vi "Plot Data.vi"(0 "Data Array":dbl[][](array[numeric]), 11 "Seconds":dbl[](array[numeric])) -> (4 "Number of Plots":i32=1, 6 "XY Plot - 1 Trace":cluster{"Seconds":dbl[], "Data Array":dbl[]}[](graph), 8 "XY Plot - 2 Traces":cluster{"Seconds":dbl[], "Data Array":dbl[]}[](graph), 10 "XY Plot - 3 Traces":cluster{"Seconds":dbl[], "Data Array":dbl[]}[](graph), 13 "XY Plot - 6 Traces":cluster{"Seconds":dbl[], "Data Array":dbl[]}[](graph), 14 "XY Plot - 5 Traces":cluster{"Seconds":dbl[], "Data Array":dbl[]}[](graph), 15 "XY Plot - 4 Traces":cluster{"Seconds":dbl[], "Data Array":dbl[]}[](graph))   [LabVIEW 2017]
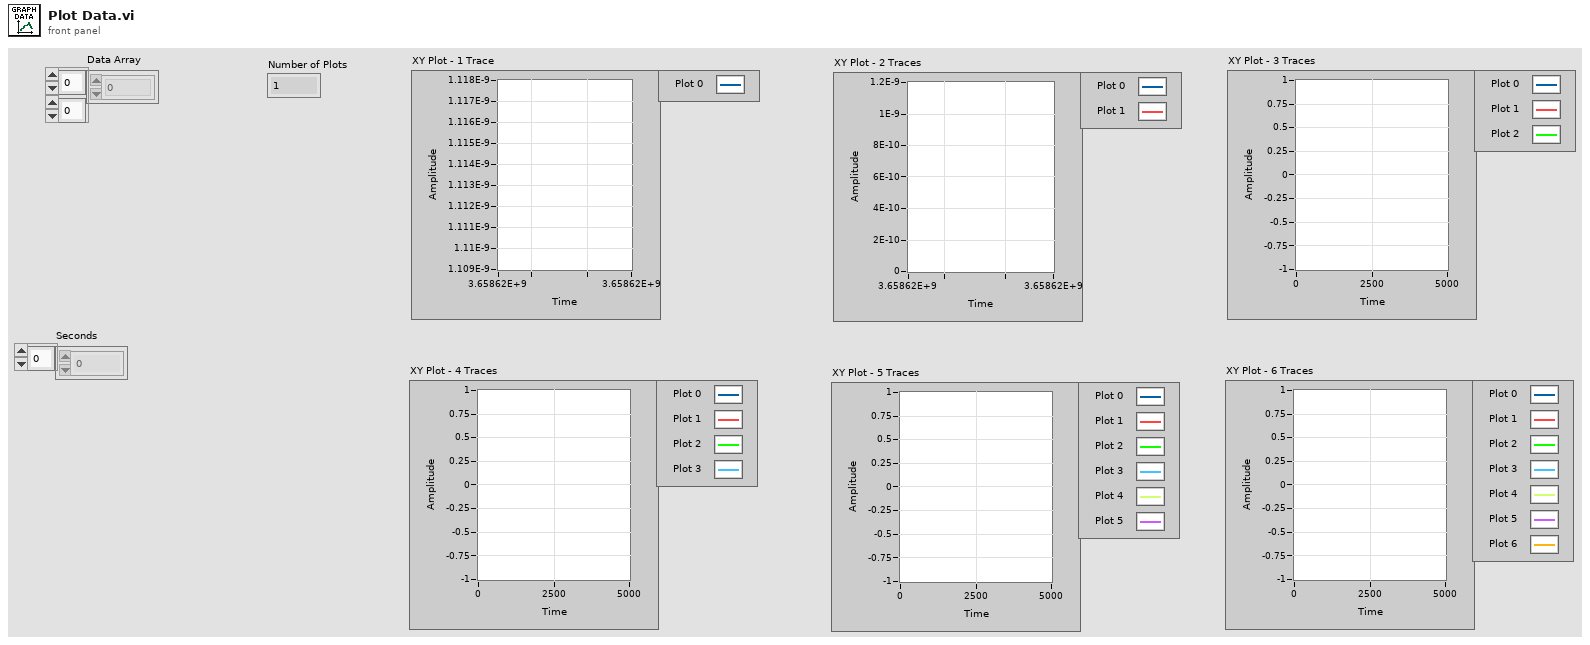
[diagram p1: front panel]
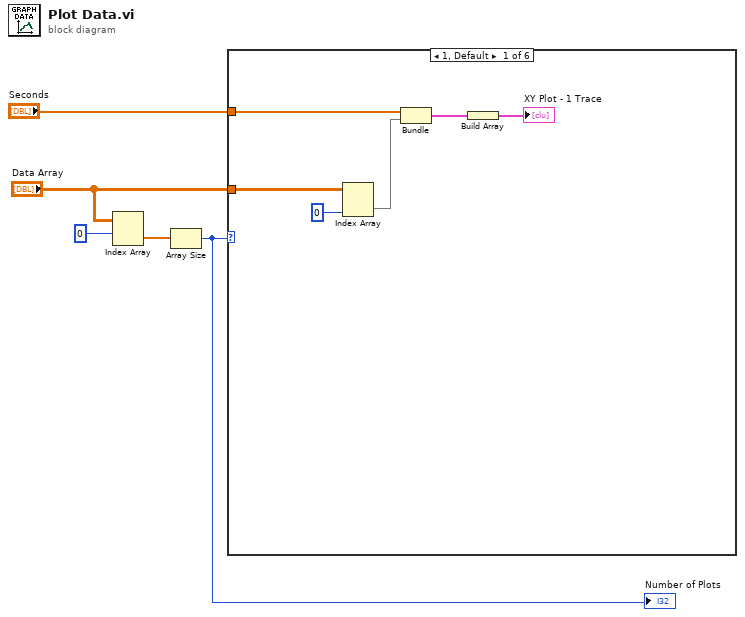
[diagram p0: block diagram]
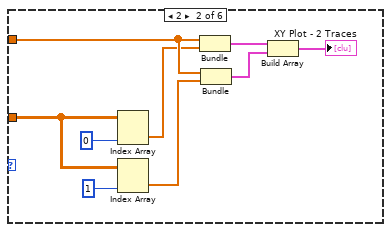
[diagram p2: hidden frame]
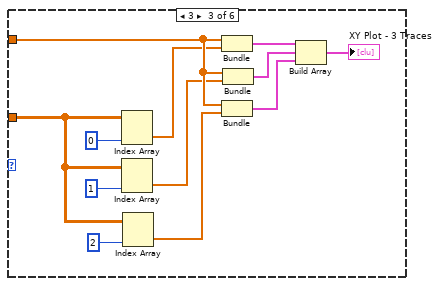
[diagram p3: hidden frame]
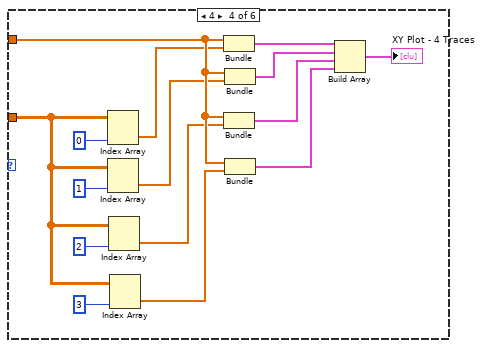
[diagram p4: hidden frame]
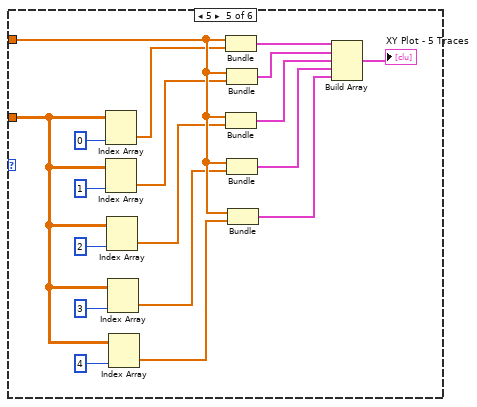
[diagram p5: hidden frame]
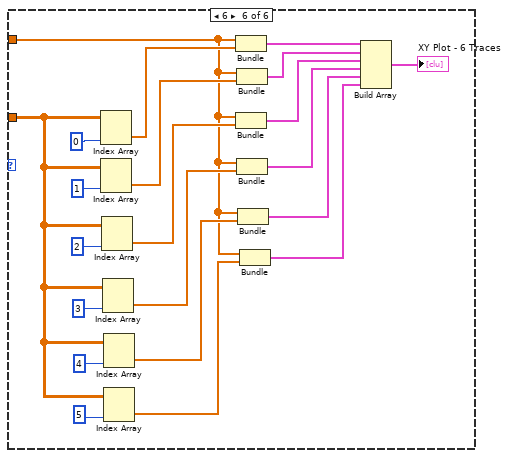
[diagram p6: hidden frame]
diagram:
  n1 = Index Array(array="Data Array", index (row)=0) -> (element=w4:dbl[])  [unwired: 1 in]
  n2 = Array Size(array=w4) -> (size(s)=w2:i32)
  "Number of Plots" <- w2
  n3 = case shown="1, Default" w2 {
    tunnel: "Seconds" -> [w11 w20 w32 w47 w65 w66]
    tunnel: "Data Array" -> [w10 w17 w25 w36 w51 w70]
    frame 1, Default {
      n4 = Index Array(array=w10, index (col)=0 ("index")) -> (element=w8:dbl[])  [unwired: 1 in]
      n5 = Bundle("Seconds"=w11, "Data Array"=w8) -> (w7:cluster{"Seconds":dbl[], "Data Array":dbl[]})  [unwired: 1 in]
      n6 = Build Array(w7) -> (→"XY Plot - 1 Trace":cluster{"Seconds":dbl[], "Data Array":dbl[]}[])
    }
    frame 2 {
      n7 = Index Array(array=w17, index (col)=0 ("index")) -> (element=w18:dbl[])  [unwired: 1 in]
      n8 = Index Array(array=w17, index (col)=1) -> (element=w15:dbl[])  [unwired: 1 in]
      n9 = Bundle("Seconds"=w20, "Data Array"=w18) -> (w14:cluster{"Seconds":dbl[], "Data Array":dbl[]})  [unwired: 1 in]
      n10 = Bundle("Seconds"=w20, "Data Array"=w15) -> (w13:cluster{"Seconds":dbl[], "Data Array":dbl[]})  [unwired: 1 in]
      n11 = Build Array(w14, w13) -> (→"XY Plot - 2 Traces":cluster{"Seconds":dbl[], "Data Array":dbl[]}[])
    }
    frame 3 {
      n12 = Index Array(array=w25, index (col)=0 ("index")) -> (element=w30:dbl[])  [unwired: 1 in]
      n13 = Index Array(array=w25, index (col)=1) -> (element=w28:dbl[])  [unwired: 1 in]
      n14 = Index Array(array=w25, index (col)=2) -> (element=w23:dbl[])  [unwired: 1 in]
      n15 = Bundle("Seconds"=w32, "Data Array"=w30) -> (w27:cluster{"Seconds":dbl[], "Data Array":dbl[]})  [unwired: 1 in]
      n16 = Bundle("Seconds"=w32, "Data Array"=w23) -> (w22:cluster{"Seconds":dbl[], "Data Array":dbl[]})  [unwired: 1 in]
      n17 = Bundle("Seconds"=w32, "Data Array"=w28) -> (w26:cluster{"Seconds":dbl[], "Data Array":dbl[]})  [unwired: 1 in]
      n18 = Build Array(w27, w26, w22) -> (→"XY Plot - 3 Traces":cluster{"Seconds":dbl[], "Data Array":dbl[]}[])
    }
    frame 4 {
      n19 = Index Array(array=w36, index (col)=0 ("index")) -> (element=w45:dbl[])  [unwired: 1 in]
      n20 = Index Array(array=w36, index (col)=1) -> (element=w43:dbl[])  [unwired: 1 in]
      n21 = Index Array(array=w36, index (col)=2) -> (element=w39:dbl[])  [unwired: 1 in]
      n22 = Index Array(array=w36, index (col)=3) -> (element=w35:dbl[])  [unwired: 1 in]
      n23 = Bundle("Seconds"=w47, "Data Array"=w45) -> (w42:cluster{"Seconds":dbl[], "Data Array":dbl[]})  [unwired: 1 in]
      n24 = Bundle("Seconds"=w47, "Data Array"=w39) -> (w38:cluster{"Seconds":dbl[], "Data Array":dbl[]})  [unwired: 1 in]
      n25 = Bundle("Seconds"=w47, "Data Array"=w43) -> (w41:cluster{"Seconds":dbl[], "Data Array":dbl[]})  [unwired: 1 in]
      n26 = Bundle("Seconds"=w47, "Data Array"=w35) -> (w34:cluster{"Seconds":dbl[], "Data Array":dbl[]})  [unwired: 1 in]
      n27 = Build Array(w42, w41, w38, w34) -> (→"XY Plot - 4 Traces":cluster{"Seconds":dbl[], "Data Array":dbl[]}[])
    }
    frame 5 {
      n28 = Index Array(array=w51, index (col)=0 ("index")) -> (element=w63:dbl[])  [unwired: 1 in]
      n29 = Index Array(array=w51, index (col)=1) -> (element=w61:dbl[])  [unwired: 1 in]
      n30 = Index Array(array=w51, index (col)=2) -> (element=w57:dbl[])  [unwired: 1 in]
      n31 = Index Array(array=w51, index (col)=3) -> (element=w54:dbl[])  [unwired: 1 in]
      n32 = Index Array(array=w51, index (col)=4) -> (element=w50:dbl[])  [unwired: 1 in]
      n33 = Bundle("Seconds"=w65, "Data Array"=w63) -> (w60:cluster{"Seconds":dbl[], "Data Array":dbl[]})  [unwired: 1 in]
      n34 = Bundle("Seconds"=w65, "Data Array"=w57) -> (w56:cluster{"Seconds":dbl[], "Data Array":dbl[]})  [unwired: 1 in]
      n35 = Bundle("Seconds"=w65, "Data Array"=w61) -> (w59:cluster{"Seconds":dbl[], "Data Array":dbl[]})  [unwired: 1 in]
      n36 = Bundle("Seconds"=w65, "Data Array"=w54) -> (w53:cluster{"Seconds":dbl[], "Data Array":dbl[]})  [unwired: 1 in]
      n37 = Bundle("Seconds"=w65, "Data Array"=w50) -> (w49:cluster{"Seconds":dbl[], "Data Array":dbl[]})  [unwired: 1 in]
      n38 = Build Array(w60, w59, w56, w53, w49) -> (→"XY Plot - 5 Traces":cluster{"Seconds":dbl[], "Data Array":dbl[]}[])
    }
    frame 6 {
      n39 = Index Array(array=w70, index (col)=0 ("index")) -> (element=w85:dbl[])  [unwired: 1 in]
      n40 = Index Array(array=w70, index (col)=1) -> (element=w83:dbl[])  [unwired: 1 in]
      n41 = Index Array(array=w70, index (col)=2) -> (element=w79:dbl[])  [unwired: 1 in]
      n42 = Index Array(array=w70, index (col)=3) -> (element=w76:dbl[])  [unwired: 1 in]
      n43 = Index Array(array=w70, index (col)=4) -> (element=w74:dbl[])  [unwired: 1 in]
      n44 = Index Array(array=w70, index (col)=5) -> (element=w68:dbl[])  [unwired: 1 in]
      n45 = Bundle("Seconds"=w66, "Data Array"=w85) -> (w82:cluster{"Seconds":dbl[], "Data Array":dbl[]})  [unwired: 1 in]
      n46 = Bundle("Seconds"=w66, "Data Array"=w79) -> (w78:cluster{"Seconds":dbl[], "Data Array":dbl[]})  [unwired: 1 in]
      n47 = Bundle("Seconds"=w66, "Data Array"=w83) -> (w81:cluster{"Seconds":dbl[], "Data Array":dbl[]})  [unwired: 1 in]
      n48 = Bundle("Seconds"=w66, "Data Array"=w76) -> (w75:cluster{"Seconds":dbl[], "Data Array":dbl[]})  [unwired: 1 in]
      n49 = Bundle("Seconds"=w66, "Data Array"=w74) -> (w73:cluster{"Seconds":dbl[], "Data Array":dbl[]})  [unwired: 1 in]
      n50 = Bundle("Seconds"=w66, "Data Array"=w68) -> (w67:cluster{"Seconds":dbl[], "Data Array":dbl[]})  [unwired: 1 in]
      n51 = Build Array(w82, w81, w78, w75, w73, w67) -> (→"XY Plot - 6 Traces":cluster{"Seconds":dbl[], "Data Array":dbl[]}[])
    }
  }
